vi "FPGA Main1.vi"() -> ()   [LabVIEW 2017]
uses:
  <vilib>/LabVIEW Targets/FPGA/cRIO/shared/nicrio_ModuleControls/nicrio_cRIO-9234_DataRatesRing2.ctl
  controls/FPGA State.ctl
  <vilib>/LabVIEW Targets/FPGA/cRIO/shared/nicrio_ModuleControls/nicrio_cRIO-9234_ConfigModeRing.ctl
  <vilib>/rvi/eio/common/nirviEmuTemplatePropertySet_noerrors.vi
  <vilib>/rvi/DataTransferAndStorage/Container/Common/niFpgaContainerGetUniqueNameForEmu.vi
  <vilib>/rvi/DataTransferAndStorage/Container/Common/niFpgaContainerSetEmuInfo.vi
  <vilib>/rvi/eio/common/nirviEmuReportErrorAndStop.vi
  <vilib>/rvi/Emulation/niFpgaEmulationIsFPGAContextNoSignature.vi
  <vilib>/rvi/Memory/Memory_Emulation/niFpgaMemoryEmulationCacheClearOnFirstRun.vi
  <vilib>/rvi/Memory/Memory_Emulation/nirvimemoryEmulationManagerCache_MakeExclusive.vi
  <vilib>/rvi/Memory/Memory_Emulation/niFpgaMemoryEmulationValidateCache.vi
  <vilib>/rvi/Memory/Memory_Emulation/nirvimemoryEmulationManagerCache_InsertValue.vi
  <vilib>/Utility/error.llb/Clear Errors.vi
  <vilib>/rvi/Memory/Memory_Emulation/nirvimemoryEmulationManagerCache_ReleaseExclusive.vi
  <vilib>/rvi/Memory/Memory_Emulation/nirvimemoryEmulationManagerCache_GetValue.vi
  <vilib>/rvi/Memory/Memory_Emulation/nirvimemoryEmulationManagerCache_SetValue.vi
  <vilib>/rvi/Emulation/niFpgaProcessEmulError.vi
  <vilib>/rvi/Emulation/niFpgaSctlEmulationGetInTimedLoop.vi
  <vilib>/rvi/eio/common/nirviEmuTemplatePropertyGet_noerrors.vi
  <vilib>/rvi/eio/common/nirviEmuTemplateMethod_errors.vi
  <vilib>/rvi/Emulation/niFpgaGetClockAttributes.vi
  <vilib>/rvi/Emulation/niFpgaEmulationReportErrorSimple.vi
  <vilib>/rvi/interface/RandomDataEmulation/niFpgaRandomDataHandleErrors.vi
  <vilib>/rvi/Emulation/niFpgaCriticalErrorInLSC.vi
  <vilib>/eio/EIOPropertyNode/EIOPropertyNode.xnode
  <vilib>/rvi/LocalResourceManager/LocalResourceManager.xnode
  <vilib>/rvi/DataTransferAndStorage/Container/XNode/niFpgaContainer.xnode
  <vilib>/rvi/DataTransferAndStorage/Register/Emulation/niFpgaRegisterEmulation.vi
  <vilib>/LabVIEW Targets/FPGA/cRIO/shared/nicrio_ModuleControls/nicrio_cRIO-9236_DataRatesRing.ctl
  <vilib>/eio/EIONode/EIONode.xnode
  <vilib>/rvi/interface/RandomDataEmulation/nirviRandomDataFpgaReadWriteTemplate.vi
  <vilib>/rvi/eio/common/nirviEmuTemplatePropertyGet_errors.vi
  <vilib>/rvi/eio/common/nirviEmuTemplatePropertySet_errors.vi
panel:
  out "Strain 8":cluster{"LSB Weight":u16, "Offset":i16}
  out "Strain 7":cluster{"LSB Weight":u16, "Offset":i16}
  out "Strain 6":cluster{"LSB Weight":u16, "Offset":i16}
  out "Strain 5":cluster{"LSB Weight":u16, "Offset":i16}
  out "Strain 4":cluster{"LSB Weight":u16, "Offset":i16}
  out "Strain 3":cluster{"LSB Weight":u16, "Offset":i16}
  out "Strain 2":cluster{"LSB Weight":u16, "Offset":i16}
  out "Strain1":cluster{"LSB Weight":u16, "Offset":i16}
  out "Acceleration Z (g)":sgl
  out "Acceleration Y (g)":sgl
  in  "Requested PID Loop Period (us)":u32=200
  out "Input Error":bool
  in  "Enable Watchdog":bool
  in  "Pet Watchdog":bool
  in  "Watchdog Timeout Period (ticks)":u64=40000000 format="%.0p"
  out "Watchdog Timed Out?":bool=TRUE
  out "Time Since Last Pet":u64
  in  "Change State":bool
  out "Current FPGA State":T1
  in  "New FPGA State":T1
  out "PID Loop Period (tick)":u32
  out "DMA FIFO Overflow?":bool
  out "Acceleration X (g)":sgl
  in  "Max Acceleration Threshold (g)":sgl=0.75
  out "Max Acceleration Exceeded?":bool
  in  "Data Rate":T2=5 items=["51.200 kS/s (NI 9234)"=1, "25.600 kS/s (NI 9234)"=2, "17.067 kS/s (NI 9234)"=3, "12.800 kS/s (NI 9234)"=4, "10.240 kS/s (NI 9234)"=5, "8.533 kS/s (NI 9234)"=6, "7.314 kS/s (NI 9234)"=7, "6.400 kS/s (NI 9234)"=8, "5.689 kS/s (NI 9234)"=9, "5.120 kS/s (NI 9234)"=10, "4.654 kS/s (NI 9234)"=11, "4.267 kS/s (NI 9234)"=12, "3.938 kS/s (NI 9234)"=13, "3.657 kS/s (NI 9234)"=14, "3.413 kS/s (NI 9234)"=15, "3.200 kS/s (NI 9234)"=16, "3.012 kS/s (NI 9234)"=17, "2.845 kS/s (NI 9234)"=18, "2.695 kS/s (NI 9234)"=19, "2.560 kS/s (NI 9234)"=20, "2.438 kS/s (NI 9234)"=21, "2.328 kS/s (NI 9234)"=22, "2.226 kS/s (NI 9234)"=23, "2.133 kS/s (NI 9234)"=24, "2.048 kS/s (NI 9234)"=25, "1.969 kS/s (NI 9234)"=26, "1.896 kS/s (NI 9234)"=27, "1.829 kS/s (NI 9234)"=28, "1.765 kS/s (NI 9234)"=29, "1.707 kS/s (NI 9234)"=30, "1.652 kS/s (NI 9234)"=31]
  out "Acquisition Loop Period (tick)":u32
  # "General Settings"
  # "Fan Speed PID Settings"
  # "Monitoring Values"
  # "General"
  # "Acceleration"
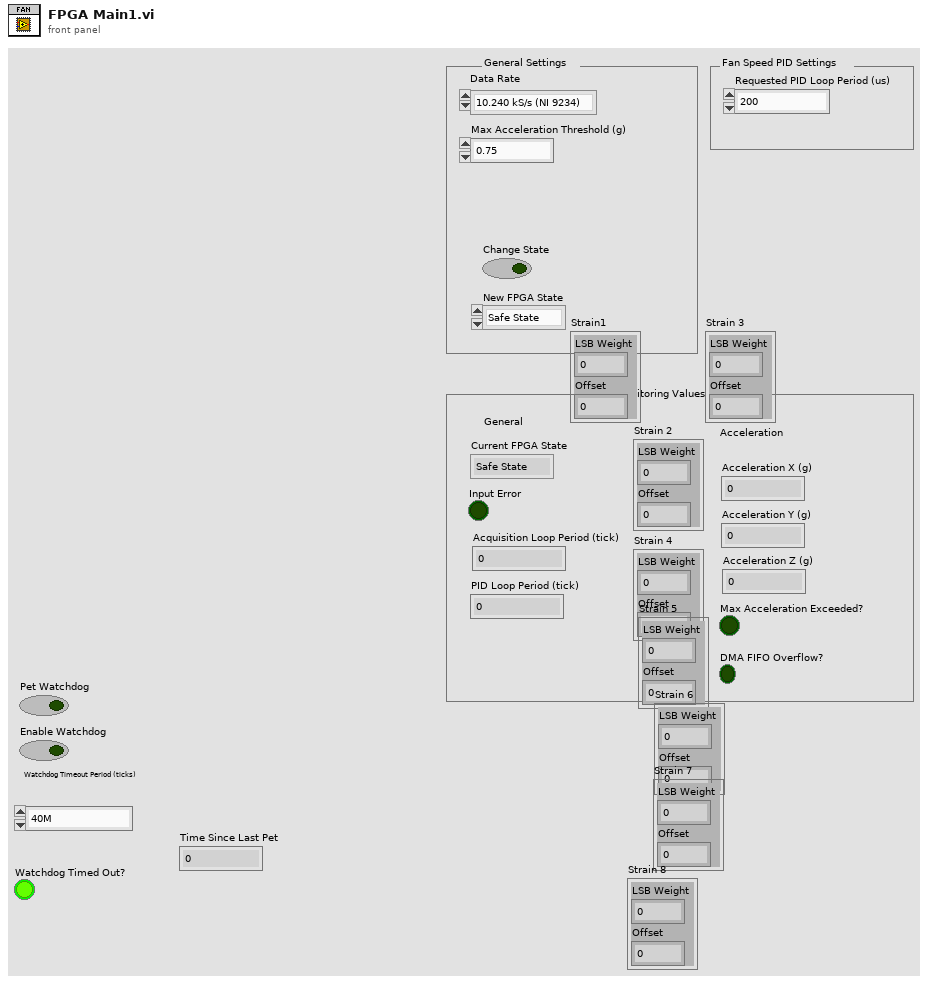
[diagram p1: front panel]
types:
  T1 = typedef "FPGA state.ctl" = enum16{"Safe State", "Control (PID)"}
  T2 = typedef "nicrio_cRIO-9234_DataRatesRing2.ctl" = u8
  T3 = typedef "nicrio_cRIO-9234_ConfigModeRing.ctl" = u8
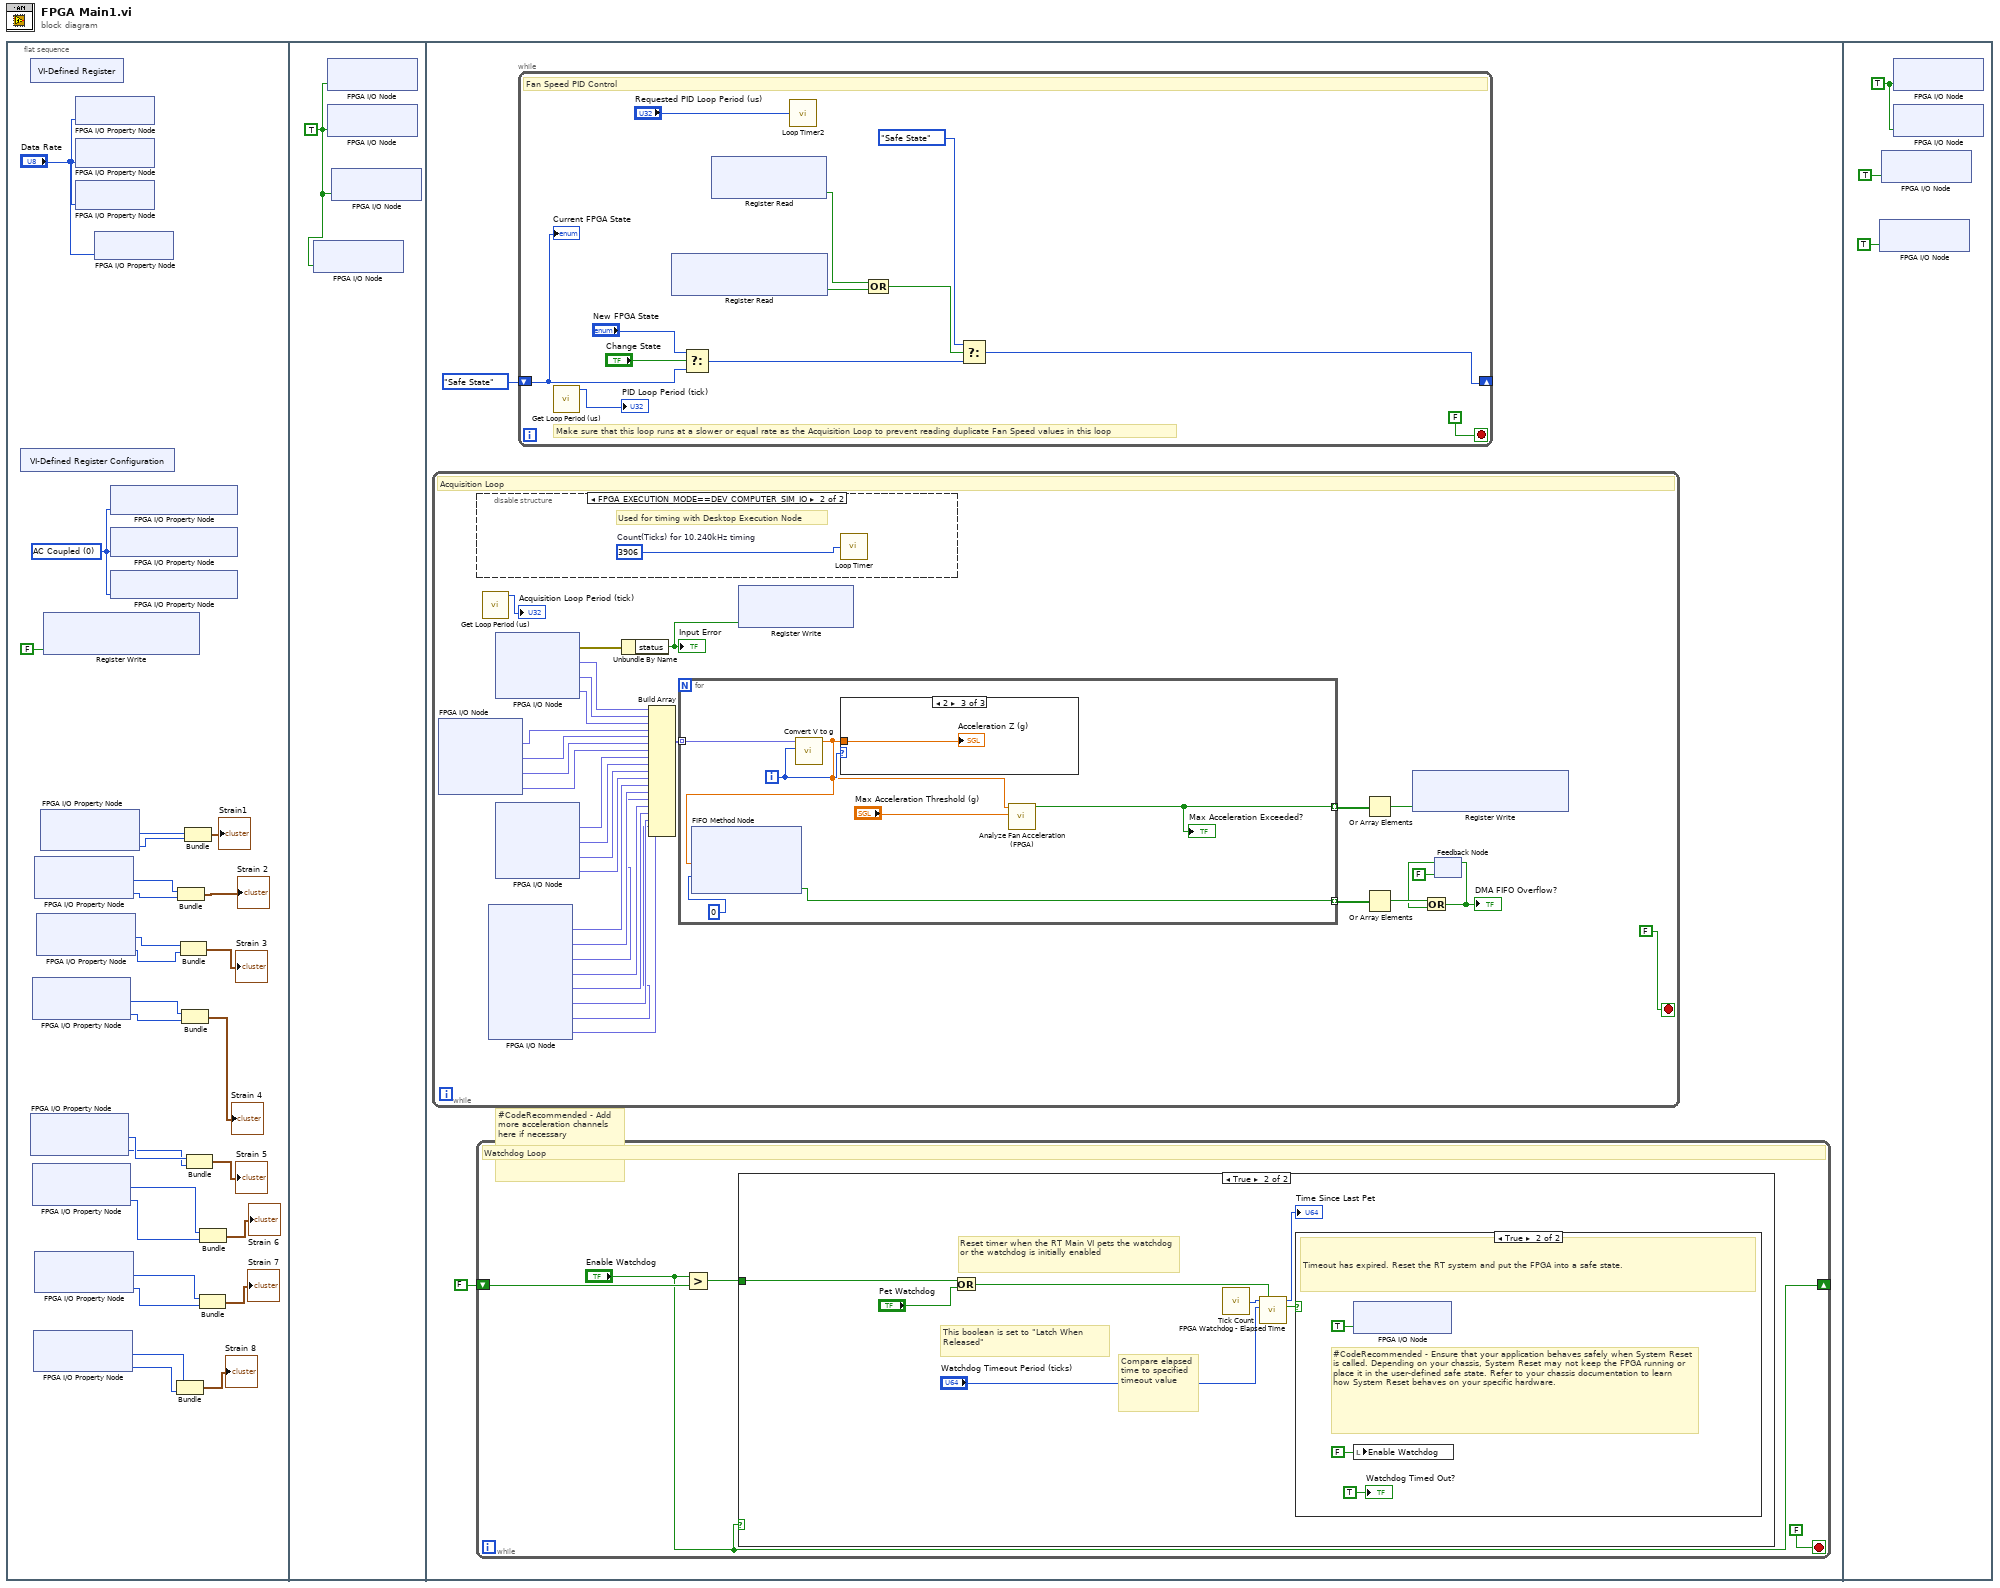
[diagram p0: block diagram]
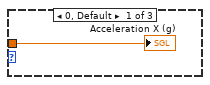
[diagram p4: hidden frame]
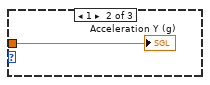
[diagram p5: hidden frame]
diagram:
  n1 = flat-sequence {
    frame #0 {
      w26 = T3 0 items=["AC Coupled", "DC Coupled", "IEPE AC Coupled"] ("Input Configuration")
      n2 = xnode ("VI-Defined Register Configuration")() -> ()  [unwired: 1 out]
      n3 = xnode "VI-Defined Register"() -> ()  [unwired: 1 out]
      n4 = xnode "FPGA I/O Property Node"() -> ("LSB Weight"=w11:u16, "Offset"=w10:i16)  [unwired: 1 in, 1 out]
      n5 = xnode "FPGA I/O Property Node"() -> ("LSB Weight"=w17:u16, "Offset"=w18:i16)  [unwired: 1 in, 1 out]
      n6 = xnode "FPGA I/O Property Node"() -> ("LSB Weight"=w7:u16, "Offset"=w8:i16)  [unwired: 1 in, 1 out]
      n7 = xnode "FPGA I/O Property Node"() -> ("LSB Weight"=w1:u16, "Offset"=w2:i16)  [unwired: 1 in, 1 out]
      n8 = xnode "FPGA I/O Property Node"() -> ("LSB Weight"=w22:u16, "Offset"=w21:i16)  [unwired: 1 in, 1 out]
      n9 = xnode "FPGA I/O Property Node"() -> ("LSB Weight"=w4:u16, "Offset"=w5:i16)  [unwired: 1 in, 1 out]
      n10 = xnode "FPGA I/O Property Node"() -> ("LSB Weight"=w20:u16, "Offset"=w19:i16)  [unwired: 1 in, 1 out]
      n11 = xnode "FPGA I/O Property Node"() -> ("LSB Weight"=w24:u16, "Offset"=w23:i16)  [unwired: 1 in, 1 out]
      n12 = xnode ("Register Write")("Data"=FALSE) -> ()  [unwired: 1 in, 1 out]
      n13 = xnode "FPGA I/O Property Node"("Data Rate"="Data Rate") -> ()  [unwired: 1 in, 1 out]
      n14 = xnode "FPGA I/O Property Node"("Data Rate"="Data Rate") -> ()  [unwired: 1 in, 1 out]
      n15 = xnode "FPGA I/O Property Node"("Data Rate"="Data Rate") -> ()  [unwired: 1 in, 1 out]
      n16 = xnode "FPGA I/O Property Node"("Data Rate"="Data Rate") -> ()  [unwired: 1 in, 1 out]
      n17 = xnode "FPGA I/O Property Node"("Input Configuration"=w26) -> ()  [unwired: 1 in, 1 out]
      n18 = xnode "FPGA I/O Property Node"("Input Configuration"=w26) -> ()  [unwired: 1 in, 1 out]
      n19 = xnode "FPGA I/O Property Node"("Input Configuration"=w26) -> ()  [unwired: 1 in, 1 out]
      n20 = Bundle("LSB Weight"=w1, "Offset"=w2) -> (→"Strain 8":cluster{"LSB Weight":u16, "Offset":i16})  [unwired: 1 in]
      n21 = Bundle("LSB Weight"=w22, "Offset"=w21) -> (→"Strain 2":cluster{"LSB Weight":u16, "Offset":i16})  [unwired: 1 in]
      n22 = Bundle("LSB Weight"=w20, "Offset"=w19) -> (→"Strain 3":cluster{"LSB Weight":u16, "Offset":i16})  [unwired: 1 in]
      n23 = Bundle("LSB Weight"=w17, "Offset"=w18) -> (→"Strain 4":cluster{"LSB Weight":u16, "Offset":i16})  [unwired: 1 in]
      n24 = Bundle("LSB Weight"=w24, "Offset"=w23) -> (→"Strain1":cluster{"LSB Weight":u16, "Offset":i16})  [unwired: 1 in]
      n25 = Bundle("LSB Weight"=w11, "Offset"=w10) -> (→"Strain 5":cluster{"LSB Weight":u16, "Offset":i16})  [unwired: 1 in]
      n26 = Bundle("LSB Weight"=w4, "Offset"=w5) -> (→"Strain 7":cluster{"LSB Weight":u16, "Offset":i16})  [unwired: 1 in]
      n27 = Bundle("LSB Weight"=w7, "Offset"=w8) -> (→"Strain 6":cluster{"LSB Weight":u16, "Offset":i16})  [unwired: 1 in]
    }
    frame #1 {
      w28 = TRUE ("Mod1/Start")
      n28 = xnode "FPGA I/O Node"("Mod4/Start"=w28) -> ()  [unwired: 1 in, 1 out]
      n29 = xnode "FPGA I/O Node"("Mod1/Start"=w28) -> ()  [unwired: 1 in, 1 out]
      n30 = xnode "FPGA I/O Node"("Mod2/Start"=w28) -> ()  [unwired: 1 in, 1 out]
      n31 = xnode "FPGA I/O Node"("Mod3/Start"=w28) -> ()  [unwired: 1 in, 1 out]
    }
    frame #2 {
      # "#CodeRecommended - Add more acceleration channels here if necessary"
      n32 = while {
        stop <- FALSE stop-if-true
        # "Acquisition Loop"
        n33 = xnode "FPGA I/O Node"() -> ("Mod2/AI0"=w56:fxp<+/-,24,4>, "Mod2/AI1"=w55:fxp<+/-,24,4>, "Mod2/AI2"=w54:fxp<+/-,24,4>, "Mod2/AI3"=w53:fxp<+/-,24,4>)  [unwired: 4 in, 4 out]
        n34 = disable-structure shown="FPGA_EXECUTION_MODE==DEV_COMPUTER_SIM_IO" {
          frame condition #0 {
          }
          frame condition #1 (active) {
            w86 = u32 3906  # Count(Ticks) for 10.240kHz timing
            # "Used for timing with Desktop Execution Node"
            n35 = call "Loop Timer"("Count(Ticks)"=w86) -> ()  [unwired: 1 out]
          }
        }
        n36 = call "Get Loop Period (us).vi"() -> ("Loop Period (us)"=→"Acquisition Loop Period (tick)":u32)  [unwired: 11 in]
        n37 = xnode "FPGA I/O Node"() -> ("Mod4/AI0"=w52:fxp<+/-,24,-4>, "Mod4/AI1"=w51:fxp<+/-,24,-4>, "Mod4/AI2"=w50:fxp<+/-,24,-4>, "Mod4/AI3"=w49:fxp<+/-,24,-4>, "Mod4/AI4"=w48:fxp<+/-,24,-4>, "Mod4/AI5"=w47:fxp<+/-,24,-4>, "Mod4/AI6"=w46:fxp<+/-,24,-4>, "Mod4/AI7"=w45:fxp<+/-,24,-4>)  [unwired: 8 in, 8 out]
        n38 = xnode "FPGA I/O Node"() -> ("error out"=w72:errorcluster, "Mod1/AI0"=w66:fxp<+/-,24,4>, "Mod1/AI1"=w65:fxp<+/-,24,4>, "Mod1/AI2"=w64:fxp<+/-,24,4>)  [unwired: 4 in, 3 out]
        n39 = xnode "FPGA I/O Node"() -> ("Mod3/AI0"=w60:fxp<+/-,24,4>, "Mod3/AI1"=w59:fxp<+/-,24,4>, "Mod3/AI2"=w58:fxp<+/-,24,4>, "Mod3/AI3"=w57:fxp<+/-,24,4>)  [unwired: 4 in, 4 out]
        n40 = Unbundle By Name(w72) -> ("status"=w71:bool)
        "Input Error" <- w71
        n41 = Build Array(w66, w65, w64, w56, w55, w54, w53, w60, w59, w58, w57, w52, w51, w50, w49, w48, w47, w46, w45) -> (w61:fxp<+/-,32,4>[])
        n42 = for {
          tunnel: w61 -> [w79] mode=indexing
          tunnel: [w81] -> w63 mode=indexing
          tunnel: [w77] -> w62 mode=indexing
          i -> [w80]
          n43 = call "Convert V to g.vi"("channel"=w80, "Accelerometer Voltage (V)"=w79) -> ("Acceleration (g)"=w78:sgl)  [unwired: 9 in]
          n44 = xnode ("FIFO Method Node")("Element"=w78, "Timeout"=0) -> ("Timed Out?"=w77:bool)  [unwired: 1 in, 1 out]
          n45 = case shown="2" w80 {
            tunnel: w78 -> [w83 w84 w85]
            frame 0, Default {
              "Acceleration X (g)" <- w83
            }
            frame 1 {
              "Acceleration Y (g)" <- w84
            }
            frame 2 {
              "Acceleration Z (g)" <- w85
            }
          }
          n46 = call "Analyze Fan Acceleration (FPGA).vi"("max acceleration threshold (g)"="Max Acceleration Threshold (g)", "acceleration (g)"=w78) -> ("max acceleration exceeded?"=w81:bool)  [unwired: 9 in]
          "Max Acceleration Exceeded?" <- w81
        }
        n47 = xnode ("Register Write")("Data"=w71) -> ()  [unwired: 1 in, 1 out]
        n48 = Or Array Elements(Boolean array=w63) -> (logical OR=w73:bool)
        n49 = Or Array Elements(Boolean array=w62) -> (logical OR=w68:bool)
        n50 = xnode ("Register Write")("Data"=w73) -> ()  [unwired: 1 in, 1 out]
        n51 = feedback #1(FALSE) -> (w67:bool)
        n52 = Or(x=w68, y=w67) -> (x .or. y?=w69:bool)
        "DMA FIFO Overflow?" <- w69
        n53 = feedback-in #1(w69) -> ()
      }
      n54 = while "RT Watchdog Loop" {
        shift-right: ["Enable Watchdog"] -> _
        shift-left: FALSE ("Enable RT Watchdog") -> [w34]
        stop <- FALSE stop-if-true
        # "Watchdog Loop"
        n55 = Greater?(x="Enable Watchdog", y=w34) -> (0:w31:bool)
        n56 = case shown="True" "Enable Watchdog" {
          tunnel: w31 -> [_ w37]
          frame False {
            # "This loop has to be explicitly enabled from the RT Main VI.  This reduces the possiblity of an endless reboot cycle."
          }
          frame True {
            # "This boolean is set to \"Latch When Released\""
            # "Compare elapsed time to specified timeout value"
            # "Reset timer when the RT Main VI pets the watchdog or the watchdog is initially enabled"
            n57 = Or(x=w37, y="Pet Watchdog") -> (x .or. y?=w36:bool)
            n58 = call "Tick Count"() -> ("Tick Count(Ticks)"=w40:u32)
            n59 = call "FPGA Watchdog - Elapsed Time.vi"("Reset"=w36, "Timeout Period"="Watchdog Timeout Period (ticks)", "Current Time"=w40) -> ("Timeout"=w35:bool, "Elapsed Time"=→"Time Since Last Pet":u64)  [unwired: 7 in]
            n60 = case shown="True" w35 {
              frame False {
                # "Timeout has not expired."
              }
              frame True {
                # "#CodeRecommended - Ensure that your application behaves safely when System Reset is called. Depending on your chassis, System Reset may not keep the FPGA running or place it in the user-defined safe state. Refer to your chassis documentation to learn how System Reset behaves on your specific hardware."
                # "Timeout has expired. Reset the RT system and put the FPGA into a safe state."
                n61 = xnode "FPGA I/O Node"("System Reset"=TRUE ("RT Reset on Watchdog Failure?")) -> ()  [unwired: 1 in, 1 out]
                n62 = local write "Enable Watchdog"(FALSE ("Enable RT Watchdog")) -> ()
                "Watchdog Timed Out?" <- TRUE ("Watchdog Timed Out?")
              }
            }
          }
        }
      }
      n63 = while {
        shift-right: [w96] -> _
        shift-left: FPGA_state."Safe State" ("FPGA state") -> [w87]
        stop <- FALSE stop-if-true
        # "Make sure that this loop runs at a slower or equal rate as the Acquisition Loop to prevent reading duplicate Fan Speed values in this loop"
        # "Fan Speed PID Control"
        n64 = call "Get Loop Period (us).vi"() -> ("Loop Period (us)"=→"PID Loop Period (tick)":u32)  [unwired: 11 in]
        n65 = xnode ("Register Read")() -> ("Data"=w88:bool)  [unwired: 1 in, 1 out]
        n66 = Select(t="New FPGA State", s="Change State", f=w87) -> (s? t:f=w91:T1)
        n67 = xnode ("Register Read")() -> ("Data"=w90:bool)  [unwired: 1 in, 1 out]
        n68 = call "Loop Timer2"("Count(uSec)"="Requested PID Loop Period (us)") -> ()  [unwired: 1 out]
        n69 = Compound Arithmetic op=OR(w90, w88) -> (w97:bool)
        n70 = Select(t=FPGA_state."Safe State", s=w97, f=w91) -> (s? t:f=w96:T1)
        "Current FPGA State" <- w87
      }
    }
    frame #3 {
      w100 = TRUE ("Mod1/Stop")
      n71 = xnode "FPGA I/O Node"("Mod4/Stop"=TRUE ("Mod1/Stop")) -> ()  [unwired: 1 in, 1 out]
      n72 = xnode "FPGA I/O Node"("Mod1/Stop"=TRUE) -> ()  [unwired: 1 in, 1 out]
      n73 = xnode "FPGA I/O Node"("Mod2/Stop"=w100) -> ()  [unwired: 1 in, 1 out]
      n74 = xnode "FPGA I/O Node"("Mod3/Stop"=w100) -> ()  [unwired: 1 in, 1 out]
    }
  }
